vi "GT_lnXY.vi"(4 "synVel":dbl, 5 "Y":i32, 6 "synAcc":dbl, 7 "X":i32, 8 "VelEnd":dbl, 9 "fifo":i16, 10 "crd":i16, 11 "rtn_In":cluster{"rtn":i16, "Func":string}) -> (1 "fifo out":i16, 2 "crd out":i16, 3 "rtn_Out":cluster{"rtn":i16, "Func":string})   [LabVIEW 2014]
uses:
  VC6/gts.dll
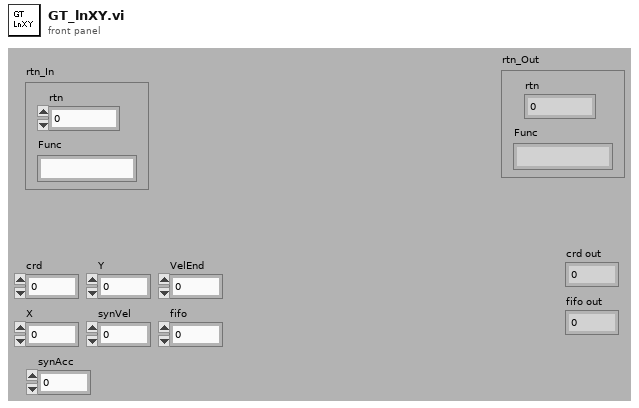
[diagram p1: front panel]
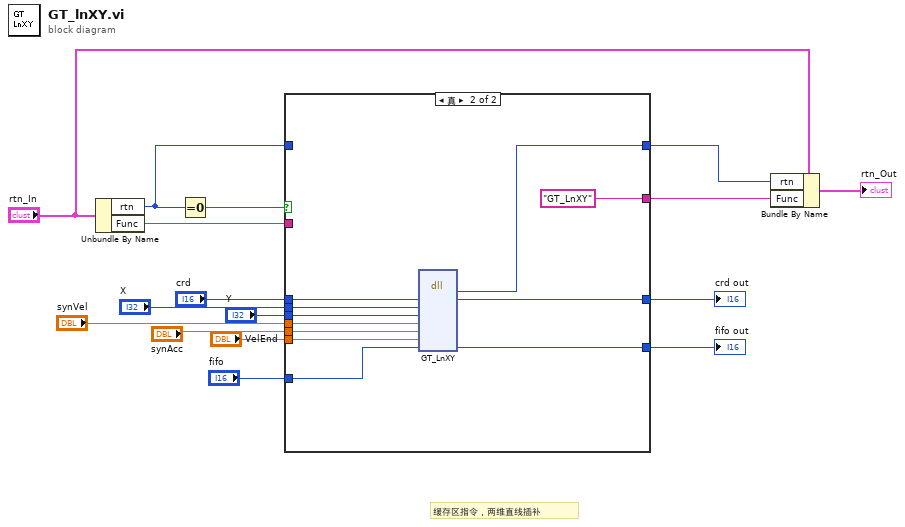
[diagram p0: block diagram]
diagram:
  # "缓存区指令，两维直线插补"
  n1 = Unbundle By Name("rtn_In") -> ("rtn"=w12:i16, "Func"=w10:string)
  n2 = Equal To 0?(x=w12) -> (x = 0?=w16:bool)
  n3 = case shown="真" w16 {
    tunnel: [w19 "GT_LnXY" ("Func")] -> w13
    tunnel: w12 -> [w20 _]
    tunnel: [w20 w30] -> w11
    tunnel: w10 -> [w19 _]
    tunnel: "crd" -> [w17 w29]
    tunnel: "X" -> [_ w28]
    tunnel: "Y" -> [_ w27]
    tunnel: "synVel" -> [_ w26]
    tunnel: "synAcc" -> [_ w25]
    tunnel: "VelEnd" -> [_ w24]
    tunnel: "fifo" -> [w18 w23]
    tunnel: [w17 w22] -> w2
    tunnel: [w18 w21] -> w1
    frame False {
    }
    frame True {
      n4 = dll-call lib="PTH2Fabs DNewGTS AC-800LWin7版源程序-20170926gts85VC6gts.dll" fn="GT_LnXY"("crd"=w29, "X"=w28, "Y"=w27, "synVel"=w26, "synAcc"=w25, "VelEnd"=w24, "fifo"=w23) -> ("rtn"=w30:i16, "crd"=w22:i16, "fifo"=w21:i16)  [unwired: 8 in, 2 out]
    }
  }
  "crd out" <- w2
  "fifo out" <- w1
  n5 = Bundle By Name(cluster="rtn_In", "rtn"=w11, "Func"=w13) -> (→"rtn_Out":cluster{"rtn":i16, "Func":string})
